vi "restart1.vi"(0 "error in":errorcluster, 1 "Bool Refnum":refnum<vi>) -> ()   [LabVIEW 2010]
uses:
  Global 2.vi
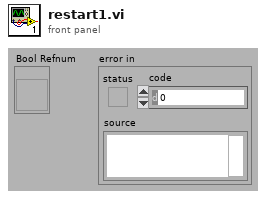
[diagram p1: front panel]
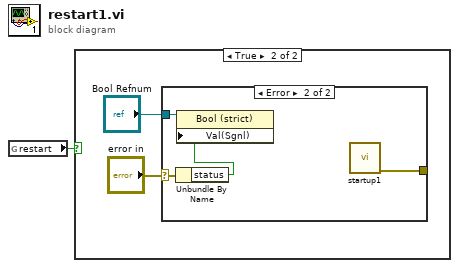
[diagram p0: block diagram]
diagram:
  n1 = global read "Global 2.vi" "restart"() -> (w1:bool)
  n2 = case shown="True" w1 {
    frame False {
    }
    frame True {
      n3 = case shown="Error" "error in" {
        selector: "error in" -> [_ w7]
        tunnel: "Bool Refnum" -> [_ w5]
        tunnel: [_ w4] -> _
        frame No Error {
        }
        frame Error {
          n4 = Unbundle By Name(w7) -> ("status"=w6:bool)
          n5 = property on="Property Node" class="Bool (strict)"(reference=w5, "Val(Sgnl)"=w6) -> ()  [unwired: 1 in, 2 out]
          n6 = call "startup1.vi"() -> ("error out"=w4:errorcluster)  [unwired: 7 in]
        }
      }
    }
  }
